vi "Read Config from File.vi"(8 "error in (no error)":errorcluster) -> (0 "error out":errorcluster, 3 "System Parameters":T1={"Optical Parameters"={"Obj. Focal Length [mm]"=0.0, "Scan Lens EFL[mm]"=0.0, "Tube Lens EFL[mm]"=0.0, "Galvo V Range (+/-)"=0.0, "Galvo Max Half Angle [Deg]"=0.0, "Max Galvo Range[%]"=0.0}, "Vibratome"={"Z Bottom [mm]"=0.0, "Pre Cut Dwell [s]"=0.0, "Blade Frequency [RPM]"=0, "Slice Speed [mm/s]"=0.0, "Post Cut Dwell [s]"=0.0, "Ramp Time [s]"=0.0, "Start X [mm]"=0.0, "Start Y [mm]"=0.0, "Slice Length [mm]"=0.0, "Slice Axis"=enum."Y Axis", "Controller VISA Ref"="COM4"}, "Table Stages"={"X Stage"={"Position"=0.0, "Is.Enabled?"=FALSE, "Is.Connected?"=FALSE, "Device SN"="45876539", "AccelerationMaximum"=0.0, "VelocityMaximum"=0.0, "Acceleration"=0.0, "Velocity"=0.0, "waitTimeout (ms)"=0, "Model"=enum."None", "Is.Homed?"=FALSE}, "Y Stage"={"Position"=0.0, "Is.Enabled?"=FALSE, "Is.Connected?"=FALSE, "Device SN"="45876539", "AccelerationMaximum"=0.0, "VelocityMaximum"=0.0, "Acceleration"=0.0, "Velocity"=0.0, "waitTimeout (ms)"=0, "Model"=enum."None", "Is.Homed?"=FALSE}, "Z Stage"={"Position"=0.0, "Is.Enabled?"=FALSE, "Is.Connected?"=FALSE, "Device SN"="45876539", "AccelerationMaximum"=0.0, "VelocityMaximum"=0.0, "Acceleration"=0.0, "Velocity"=0.0, "waitTimeout (ms)"=0, "Model"=enum."None", "Is.Homed?"=FALSE}}, "Imaging Parameter"={"Raster Scan Direction"=enum."Bi Directional", "Pixel Dwell Time [Clock Cycles]"=1, "Flyback Time [Clock Cycles]"=200, "XY Center [um]"={"X"=1.0, "Y"=1.0}, "Pixel Step Size [um]"=2.5, "XY Image Size"=enum."2048 x 2048", "Custom"=FALSE, "Custom Size"={"X"=1, "Y"=1}, "Line Averages"=1}, "Galvo HW Parameters"={"Analog Out Channel"="GalvoCtrl/ao0,GalvoCtrl/ao1", "Min Voltage"=-10.0, "Max Voltage"=10.0, "Pixel Clock Source"="/GalvoCtrl/PFI0", "Sample Rate"=1000.0, "Line Clock Out Ch"="GalvoCtrl/port0/line0"}, "Alazar parameters"={"Trigger Settings"={"General Trigger Settings"={"Trigger Operation"=0, "Coupling ID"=2, "Range ID"=2, "Delay"=0, "Timeout Ticks"=0, "Mode"=1, "Parameter"=1}, "Trigger Engine 1"={"Trigger Engine"=0, "Source"=2, "Slope"=1, "Level"=140}, "Trigger Engine 2"={"Trigger Engine"=1000, "Source"=4294967295, "Slope"=1, "Level"=2048}}, "Capture Clock"={"Sample Rate"=100, "Decimation"=0, "Source"=2, "Edge"=0}, "Device ID"={"System ID"=1, "Board ID"=1}, "Ch A Input Control"={"Channel"=1, "Coupling"=2, "Range"=10, "Impedance"=2}, "Ch B Input Control"={"Channel"=2, "Coupling"=2, "Range"=10, "Impedance"=2}, "Acq Settings"={"Window Type"=1, "Record Length"=1440, "Footer"=0, "Output Format"=10, "Offset"=0, "Records Per Buffer"=2048, "Samples per record"=2048, "Records Count (Records/Acq)"=2147483647}}, "Mosaic Paramter"={"X Axis"={"Start [mm]"=0.0, "Steps [pts]"=0, "End [mm]"=0.0}, "Y Axis"={"Start [mm]"=0.0, "Steps [pts]"=0, "End [mm]"=0.0}, "Scan Pattern"=enum."Uni-directional", "Overlap Options"={"Overlap Type"=enum."No Overlap", "Percent Overlap"=0, "Justify"=enum."Start"}}} {"Alazar parameters"."Acq Settings"."Window Type" items=["DSP_WINDOW_NONE", "DSP_WINDOW_HANNING", "DSP_WINDOW_HAMMING", "DSP_WINDOW_BLACKMAN", "DSP_WINDOW_BLACKMAN_HARRIS", "DSP_WINDOW_BARTLETT"]; "Alazar parameters"."Acq Settings"."Footer" items=["FOOTER_NONE", "FOOTER_NPT"]; "Alazar parameters"."Acq Settings"."Output Format" items=["FLOAT_AMP2"=10, "FLOAT_LOG"=11]; "Alazar parameters"."Ch B Input Control"."Channel" items=["A"=1, "B"=2, "C"=4, "D"=8]; "Alazar parameters"."Ch B Input Control"."Coupling" items=["AC"=1, "DC"=2]; "Alazar parameters"."Ch B Input Control"."Range" items=["20 mV"=1, "40 mV"=2, "50 mV"=3, "80 mV"=4, "100 mV"=5, "200 mV"=6, "400 mV"=7, "500 mV"=8, "800 mV"=9, "1 V"=10, "1.25 V"=33, "2 V"=11, "4 V"=12, "5 V"=13, "8 V"=14, "10 V"=15, "20 V"=16]; "Alazar parameters"."Ch B Input Control"."Impedance" items=["1 MOhm"=1, "50 Ohm"=2, ""=0]; "Alazar parameters"."Ch A Input Control"."Channel" items=["A"=1, "B"=2, "C"=4, "D"=8]; "Alazar parameters"."Ch A Input Control"."Coupling" items=["AC"=1, "DC"=2]; "Alazar parameters"."Ch A Input Control"."Range" items=["20 mV"=1, "40 mV"=2, "50 mV"=3, "80 mV"=4, "100 mV"=5, "200 mV"=6, "400 mV"=7, "500 mV"=8, "800 mV"=9, "1 V"=10, "1.25 V"=33, "2 V"=11, "4 V"=12, "5 V"=13, "8 V"=14, "10 V"=15, "20 V"=16]; "Alazar parameters"."Ch A Input Control"."Impedance" items=["1 MOhm"=1, "50 Ohm"=2, ""=0]; "Alazar parameters"."Capture Clock"."Edge" items=["Rising", "Falling"]; "Alazar parameters"."Capture Clock"."Source" items=["Internal"=1, "Fast External"=2, "Medium External"=3, "Slow External"=4, "External AC"=5, "External DC"=6, "External 10MHz"=7]; "Alazar parameters"."Trigger Settings"."General Trigger Settings"."Trigger Operation" items=["J", "K", "J OR K", "J AND K", "J XOR K", "J AND NOT K", "NOT J AND K"]; "Alazar parameters"."Trigger Settings"."General Trigger Settings"."Coupling ID" items=["AC"=1, "DC"=2]; "Alazar parameters"."Trigger Settings"."General Trigger Settings"."Range ID" items=["5 V", "1 V", "TTL"]; "Alazar parameters"."Trigger Settings"."Trigger Engine 1"."Trigger Engine" items=["J", "K"]; "Alazar parameters"."Trigger Settings"."Trigger Engine 1"."Source" items=["A", "B", "External", "Disable", "C", "D"]; "Alazar parameters"."Trigger Settings"."Trigger Engine 1"."Slope" items=["Positive"=1, "Negative"=2]; "Alazar parameters"."Trigger Settings"."Trigger Engine 2"."Trigger Engine" items=["J", "K"]; "Alazar parameters"."Trigger Settings"."Trigger Engine 2"."Source" items=["A", "B", "External", "Disable", "C", "D"]; "Alazar parameters"."Trigger Settings"."Trigger Engine 2"."Slope" items=["Positive"=1, "Negative"=2]; "Imaging Parameter"."Line Averages" min=1 max=30 step=1; "Imaging Parameter"."Flyback Time [Clock Cycles]" max=10 step=1; "Imaging Parameter"."Pixel Step Size [um]" min=0.0 max=10.0 step=0.01; "Imaging Parameter"."Custom Size"."Y" min=1 max=30 step=1; "Imaging Parameter"."Custom Size"."X" min=1 max=30 step=1; "Imaging Parameter"."XY Center [um]"."Y" min=1.0 max=30.0 step=1.0; "Imaging Parameter"."XY Center [um]"."X" min=1.0 max=30.0 step=1.0; "Imaging Parameter"."Pixel Dwell Time [Clock Cycles]" max=10 step=1})   [LabVIEW 2018]
uses:
  Controls/System Parameters.ctl
  Controls/Optical Parameters.ctl
  Controls/Vibratome Parameters.ctl
  Controls/Translation Stage Parameters.ctl
  Hardware Mfg/Thorlabs Translation Stages/Controls/Translation Stage Cluster.ctl
  Controls/Translation Stage Types.ctl
  Controls/Imaging Parameters.ctl
  Controls/Scan Direction.ctl
  type defines/Alazar parameters.ctl
  Hardware Mfg/AlazarTech SDK/Controls/General Trigger Settings.ctl
  Hardware Mfg/AlazarTech SDK/Controls/Trigger Engine Controls.ctl
  Hardware Mfg/AlazarTech SDK/Controls/Clock Controls.ctl
  Hardware Mfg/AlazarTech SDK/Controls/Alazar Device ID.ctl
  Hardware Mfg/AlazarTech SDK/Controls/Channel Input Controls.ctl
  Hardware Mfg/AlazarTech SDK/Controls/Alazar Acquisition Settings.ctl
  <vilib>/Utility/config.llb/NI_LVConfig.lvlib
panel:
  # "X"
  # "X"
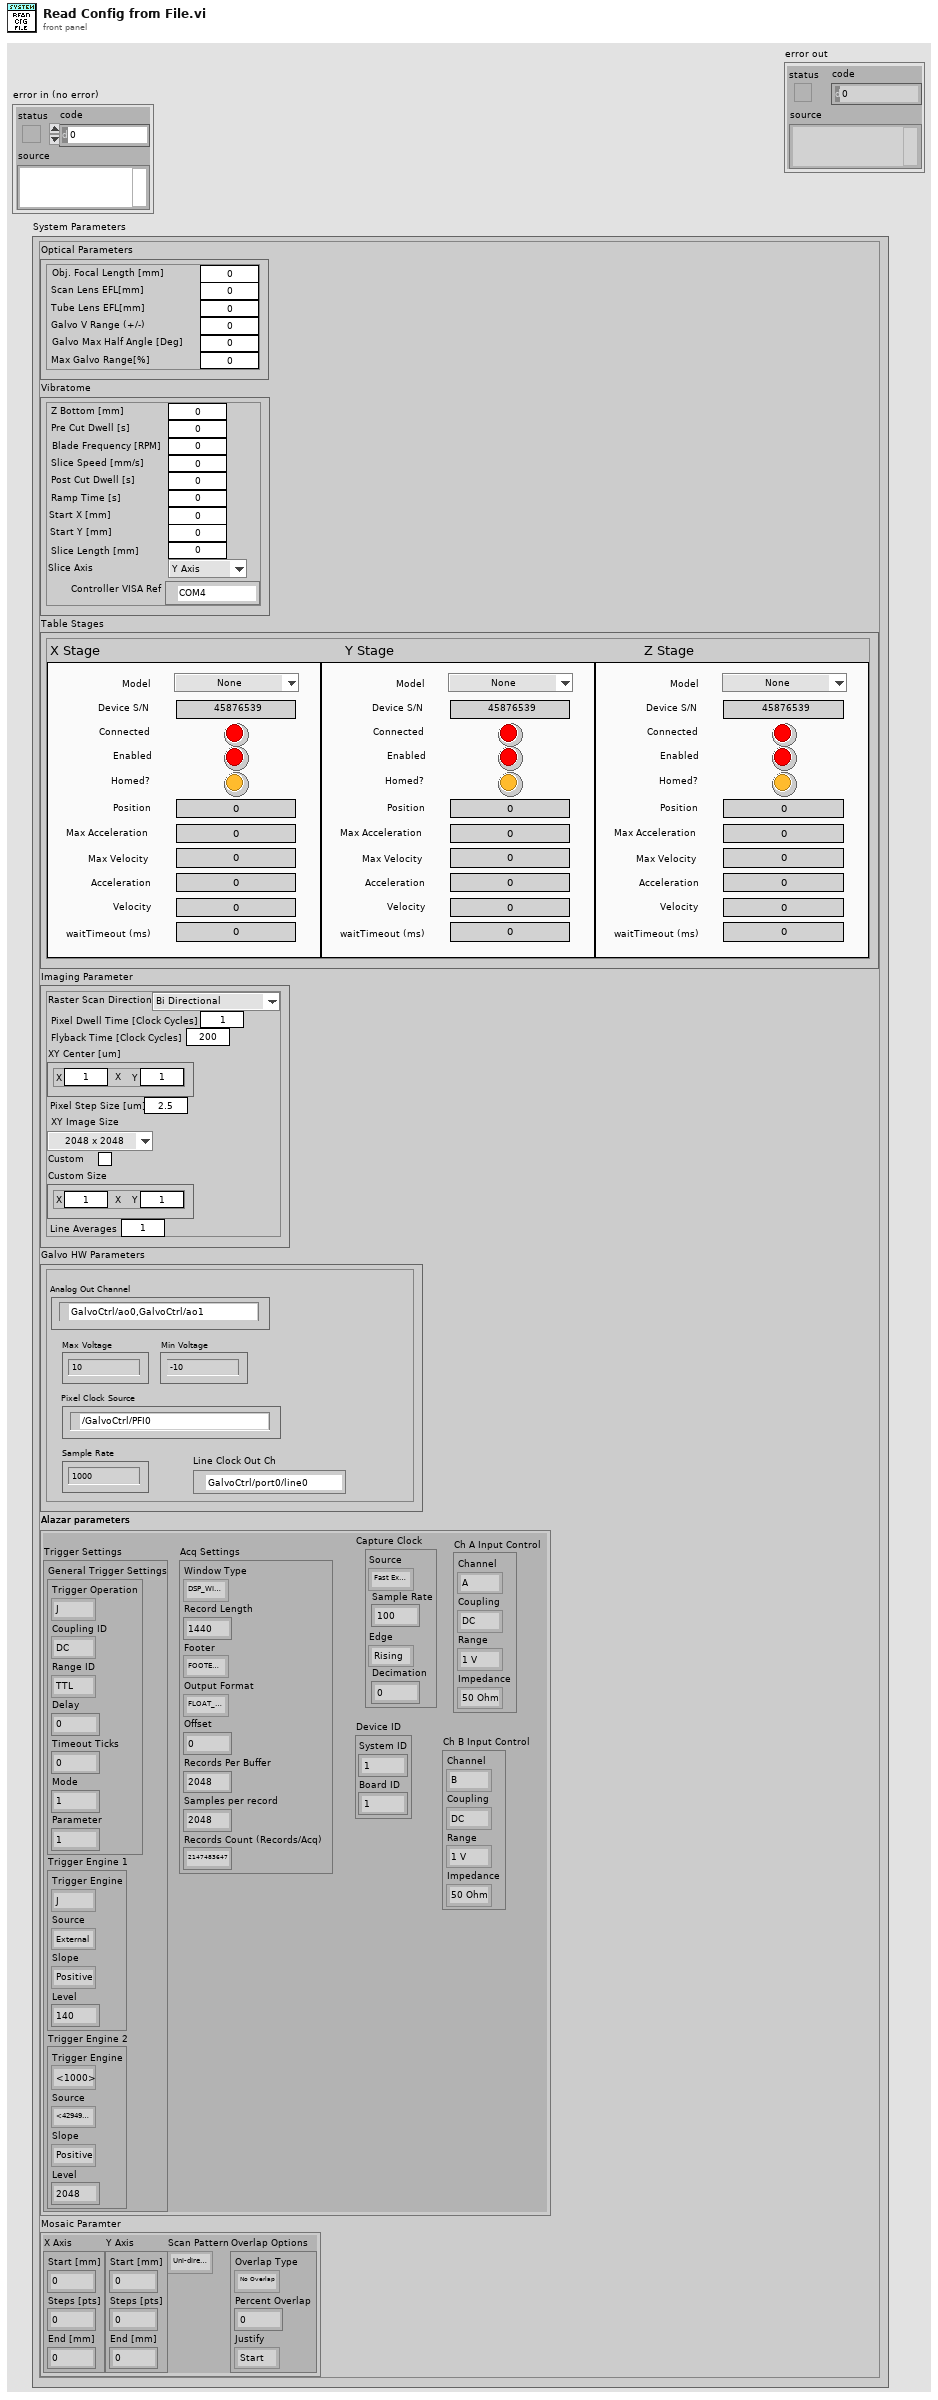
[diagram p1: front panel]
types:
  T1 = typedef "System Parameters.ctl" = cluster{"Optical Parameters":T2, "Vibratome":T3, "Table Stages":T4, "Imaging Parameter":T7, "Galvo HW Parameters":cluster{"Analog Out Channel":tag, "Min Voltage":dbl, "Max Voltage":dbl, "Pixel Clock Source":tag, "Sample Rate":dbl, "Line Clock Out Ch":tag}, "Alazar parameters":T9, "Mosaic Paramter":cluster{"X Axis":cluster{"Start [mm]":dbl, "Steps [pts]":u16, "End [mm]":dbl}, "Y Axis":cluster{"Start [mm]":dbl, "Steps [pts]":u16, "End [mm]":dbl}, "Scan Pattern":enum16{"Uni-directional", "Bi-Directional", "Spiral Out", "Spiral In"}, "Overlap Options":cluster{"Overlap Type":enum16{"No Overlap", "X Only", "Y Only", "X and Y"}, "Percent Overlap":u8, "Justify":enum16{"Start", "Center", "End"}}}}
  T2 = typedef "Optical Parameters.ctl" = cluster{"Obj. Focal Length [mm]":dbl, "Scan Lens EFL[mm]":dbl, "Tube Lens EFL[mm]":dbl, "Galvo V Range (+/-)":dbl, "Galvo Max Half Angle [Deg]":dbl, "Max Galvo Range[%]":dbl}
  T3 = typedef "Vibratome Parameters.ctl" = cluster{"Z Bottom [mm]":dbl, "Pre Cut Dwell [s]":dbl, "Blade Frequency [RPM]":u16, "Slice Speed [mm/s]":dbl, "Post Cut Dwell [s]":dbl, "Ramp Time [s]":dbl, "Start X [mm]":dbl, "Start Y [mm]":dbl, "Slice Length [mm]":dbl, "Slice Axis":enum16{"X Axis", "Y Axis", "Z Axis"}, "Controller VISA Ref":refnum<visa-resource-name>}
  T4 = typedef "Translation Stage Parameters.ctl" = cluster{"X Stage":T5, "Y Stage":T5, "Z Stage":T5}
  T5 = typedef "Translation Stage Cluster.ctl" = cluster{"Position":dbl, "Is.Enabled?":bool, "Is.Connected?":bool, "Device SN":string, "AccelerationMaximum":dbl, "VelocityMaximum":dbl, "Acceleration":dbl, "Velocity":dbl, "waitTimeout (ms)":i32, "Model":T6, "Is.Homed?":bool}
  T6 = typedef "Translation Stage Types.ctl" = enum16{"None", "Thorlabs LTS", "Thorlabs MLJ"}
  T7 = typedef "Imaging Parameters.ctl" = cluster{"Raster Scan Direction":T8, "Pixel Dwell Time [Clock Cycles]":u16, "Flyback Time [Clock Cycles]":u16, "XY Center [um]":cluster{"X":dbl, "Y":dbl}, "Pixel Step Size [um]":dbl, "XY Image Size":enum16{"32 x 32", "64 x 64", "128 x 128", "256 x 256", "512 x 512", "1024 x 1024", "2048 x 2048"}, "Custom":bool, "Custom Size":cluster{"X":u16, "Y":u16}, "Line Averages":u8}
  T8 = typedef "Scan Direction.ctl" = enum16{"Uni Directional", "Bi Directional", "None"}
  T9 = typedef "Alazar parameters.ctl" = cluster{"Trigger Settings":cluster{"General Trigger Settings":T10, "Trigger Engine 1":T11, "Trigger Engine 2":T11}, "Capture Clock":T12, "Device ID":T13, "Ch A Input Control":T14, "Ch B Input Control":T14, "Acq Settings":T15}
  T10 = typedef "General Trigger Settings.ctl" = cluster{"Trigger Operation":u32, "Coupling ID":u32, "Range ID":u32, "Delay":u32, "Timeout Ticks":u32, "Mode":u32, "Parameter":u32}
  T11 = typedef "Trigger Engine Controls.ctl" = cluster{"Trigger Engine":u32, "Source":u32, "Slope":u32, "Level":u32}
  T12 = typedef "Clock Controls.ctl" = cluster{"Sample Rate":u32, "Decimation":u32, "Source":u32, "Edge":u32}
  T13 = typedef "Alazar Device ID.ctl" = cluster{"System ID":u32, "Board ID":u32}
  T14 = typedef "Channel Input Controls.ctl" = cluster{"Channel":u8, "Coupling":u32, "Range":u32, "Impedance":u32}
  T15 = typedef "Alazar Acquisition Settings.ctl" = cluster{"Window Type":u32, "Record Length":u32, "Footer":u32, "Output Format":u32, "Offset":u32, "Records Per Buffer":u32, "Samples per record":u32, "Records Count (Records/Acq)":u32}
  T16 = typedef "NI_LVConfig.lvlib/Config Data RefNum.ctl" = refnum<k1>
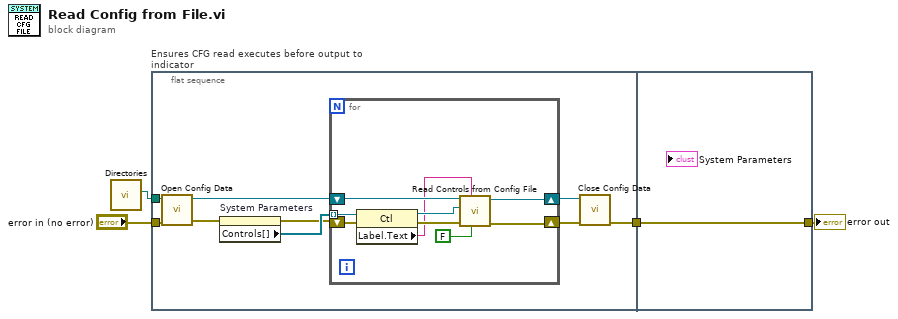
[diagram p0: block diagram]
diagram:
  n1 = call "Directories.vi"() -> ("Config.ini Path"=w2:path)  [unwired: 10 in, 1 out]
  n2 = flat-sequence "Ensures CFG read executes before output to indicator" {
    tunnel: "error in (no error)" -> [w13]
    tunnel: w2 -> [w11]
    tunnel: [w12] -> w1
    tunnel: [w23] -> w3
    tunnel: w1 -> [w23]
    frame #0 {
      n3 = call <vilib>:"Open Config Data.vi"("error in (no error)"=w13, "configuration file path"=w11) -> ("error out"=w5:errorcluster, "refnum"=w8:T16)  [unwired: 7 in, 1 out]
      n4 = property on="System Parameters" class="Clust (strict)"(error in=w5) -> (error out=w6:errorcluster, "Controls[]"=w10:refnum<vi>[])  [unwired: 1 in, 1 out]
      n5 = for {
        tunnel: w10 -> [w22] mode=indexing
        shift-right: [w18] -> w9
        shift-left: w6 -> [w21]
        shift-right: [w14] -> w7
        shift-left: w8 -> [w17]
        n6 = property class="Ctl"(reference=w22, error in=w21) -> (reference out=w16:refnum<vi>, error out=w19:errorcluster, "Label.Text"=w15:string)
        n7 = call "Read Controls from Config File.vi"("Child?"=FALSE, "section"=w15, "Error In"=w19, "Ctl Refnum"=w16, "refnum"=w17) -> ("Error Out"=w18:errorcluster, "refnum out"=w14:T16)  [unwired: 5 in]
      }
      n8 = call <vilib>:"Close Config Data.vi"("error in (no error)"=w9, "refnum"=w7) -> ("error out"=w12:errorcluster)  [unwired: 8 in, 1 out]
    }
    frame #1 {
    }
  }
  "error out" <- w3
